vi "openbci_eeg_order_8ch_16ch.vi"(10 "n_ch (8)":T1, 11 "EEG data in":dbl[][](array[numeric])) -> (3 "EEG data out":dbl[][](array[numeric]))   [LabVIEW 2013]
doc: "This VI handles the samples obtained from the OpenBCI 8ch or 16ch.\nIf 8ch, the output is an Array of [nSamples, 9 columns] 9 = 1counter + 8ch\nIf 16ch, the output is an Array of [nSamples, 17 columns] 17 = 1counter + 16ch"
uses:
  Comm Protocol/Control Def/channel_count.ctl
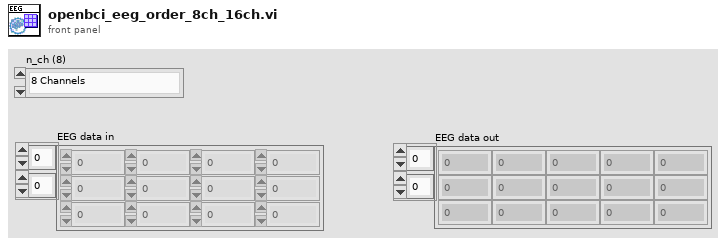
[diagram p1: front panel]
types:
  T1 = typedef "channel_count.ctl" = enum16{"8 Channels", "16 Channels"}
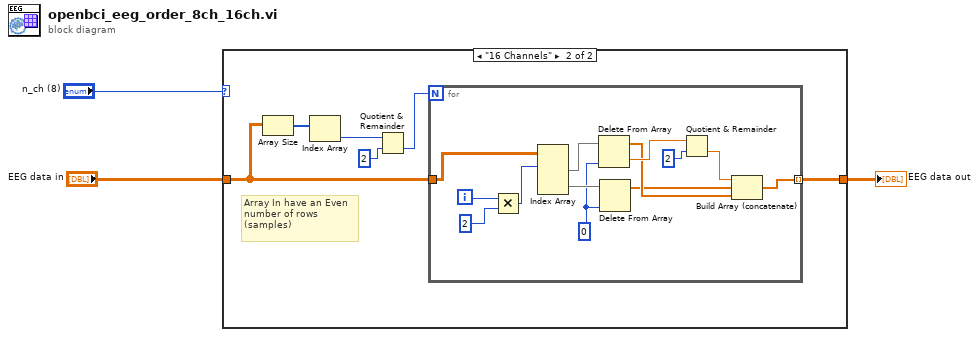
[diagram p0: block diagram]
diagram:
  n1 = case shown="\"16 Channels\"" "n_ch (8)" {
    tunnel: "EEG data in" -> [w4 w6]
    tunnel: [w4 w5] -> w3
    frame "8 Channels", Default {
    }
    frame "16 Channels" {
      # "Array In have an Even\nnumber of rows\n(samples)"
      n2 = Array Size(array=w6) -> (size(s)=w10:i32[])
      n3 = Index Array(array=w10) -> (element=w7:i32)  [unwired: 1 in]
      n4 = Quotient & Remainder(x=w7, y=2) -> (floor(x/y)=w9:i32)  [unwired: 1 out]
      n5 = for {
        N: w9 -> [_]
        tunnel: w6 -> [w21]
        tunnel: [w18] -> w5 mode=indexing
        i -> [w23]
        w17 = 0 ("index")
        n6 = Multiply(x=w23, y=2) -> (x*y=w20:i32)
        n7 = Index Array(array=w21, index (row) #1=w20) -> (element #1=w16:dbl[], element #2=w19:dbl[])  [unwired: 3 in]
        n8 = Delete From Array(array=w16, index=w17) -> (deleted portion=w13:dbl, array with subset deleted=w12:dbl[])  [unwired: 1 in]
        n9 = Delete From Array(array=w19, index=w17) -> (array with subset deleted=w11:dbl[])  [unwired: 1 in, 1 out]
        n10 = Quotient & Remainder(x=w13, y=2) -> (floor(x/y)=w14:dbl)  [unwired: 1 out]
        n11 = Build Array (concatenate)(w14, w11, w12) -> (w18:dbl[])
      }
    }
  }
  "EEG data out" <- w3
